vi "Auslesen.vi"(8 "Fehler (Eingang, kein Fehler)":errorcluster, 10 "Code":u8, 11 "VISA-Ressourcenname":refnum<visa-resource-name>) -> (0 "Fehler (Ausgang)":errorcluster, 2 "Wert":u8, 3 "VISA-Ressourcenname (Ausgang)":refnum<visa-resource-name>)   [LabVIEW 2020, in "Lambda_ Komm.lvlib"]
uses:
  Lambda_ Komm.lvlib
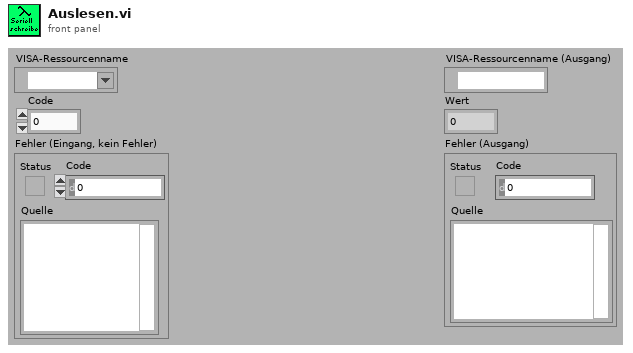
[diagram p1: front panel]
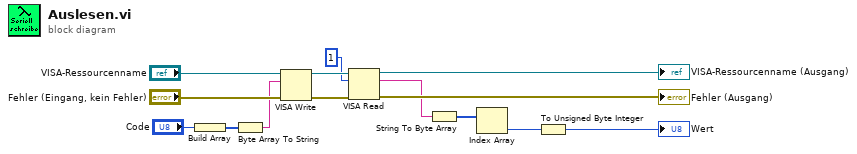
[diagram p0: block diagram]
diagram:
  n1 = Build Array("Code") -> (w6:u8[])
  n2 = Byte Array To String(unsigned byte array=w6) -> (string=w5:string)
  n3 = VISA Write(VISA resource name="VISA-Ressourcenname", write buffer=w5, error in (no error)="Fehler (Eingang, kein Fehler)") -> (VISA resource name out=w9:refnum<visa-resource-name>, error out=w7:errorcluster)  [unwired: 1 out]
  n4 = VISA Read(VISA resource name=w9, byte count=u32 1 ("Byte-Anzahl"), error in (no error)=w7) -> (VISA resource name out=→"VISA-Ressourcenname (Ausgang)":refnum<visa-resource-name>, read buffer=w4:string, error out=→"Fehler (Ausgang)":errorcluster)  [unwired: 1 out]
  n5 = String To Byte Array(string=w4) -> (unsigned byte array=w3:u8[])
  n6 = Index Array(array=w3) -> (element=w2:u8)  [unwired: 1 in]
  n7 = To Unsigned Byte Integer(number=w2) -> (unsigned 8bit integer=→"Wert":u8)
